vi "Read Com_Set.vi"(8 "error in (no error)":errorcluster, 11 "Modbus in":refnum<class "Modbus.lvclass">) -> (0 "error out":errorcluster, 2 "Com_Set":T1, 3 "Modbus out":refnum<class "Modbus.lvclass">)   [LabVIEW 2019, in "Modbus.lvclass"]
uses:
  Modbus.lvclass
  SettingCtrl.ctl
  Modbus.lvclass/Modbus.ctl
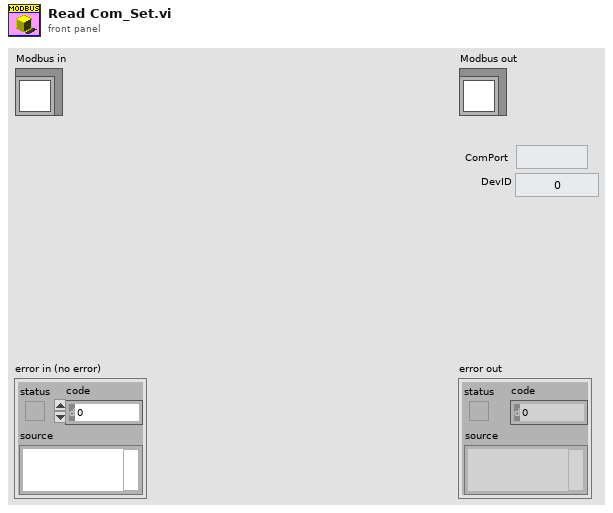
[diagram p1: front panel]
types:
  T1 = typedef "Modbus.lvclass/SettingCtrl.ctl" = cluster{"DevID":u16, "ComPort":string}
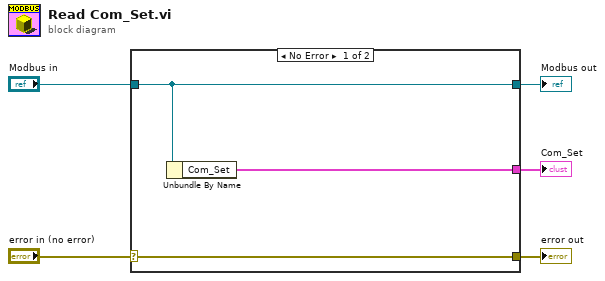
[diagram p0: block diagram]
diagram:
  n1 = case shown="No Error" "error in (no error)" {
    selector: "error in (no error)" -> [w8 w9]
    tunnel: [w8 w9] -> w4
    tunnel: [w7 w10] -> w2
    tunnel: "Modbus in" -> [w7 w10]
    tunnel: [w6 _] -> w1
    frame No Error {
      n2 = Unbundle By Name(w7) -> ("Com_Set"=w6:T1)
    }
    frame Error {
    }
  }
  "error out" <- w4
  "Modbus out" <- w2
  "Com_Set" <- w1
